vi "lsl get channel count.vi"(8 "error in (no error)":errorcluster, 11 "streaminfo":T1) -> (0 "error out":errorcluster, 3 "channel count":i32)   [LabVIEW 2018, in "liblsl-LabVIEW.lvlib"]
doc: "extern LIBLSL_C_API int32_t lsl_get_channel_count(lsl_streaminfo info);"
uses:
  <userlib>/liblsl-LabVIEW/liblsl-LabVIEW.lvlib
  <userlib>/liblsl-LabVIEW/Custom Controls/lsl_streaminfo.ctl
  <userlib>/liblsl-LabVIEW/liblsl64.dll
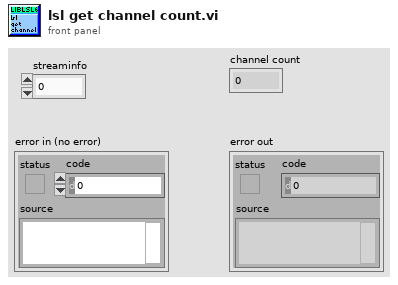
[diagram p1: front panel]
types:
  T1 = typedef "liblsl-LabVIEW.lvlib/lsl_streaminfo.ctl" = u64
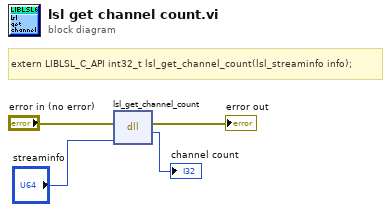
[diagram p0: block diagram]
diagram:
  # "extern LIBLSL_C_API int32_t lsl_get_channel_count(lsl_streaminfo info);"
  n1 = dll-call lib="C:/Program Files/National Instruments/LabVIEW 2018/user.lib/liblsl-LabVIEW/liblsl64.*" fn="lsl_get_channel_count"(error in="error in (no error)", "info"="streaminfo") -> (error out=→"error out":errorcluster, "return type"=→"channel count":i32)  [unwired: 3 in, 1 out]
